vi "Read Target to Host FIFO.vi"(8 "error in (no error)":errorcluster) -> (0 "error out":errorcluster, 3 "Target to Host Data":u64[](array[numeric]))   [LabVIEW 2016]
uses:
  Host/Typedefs/IO Buffer Operation.ctl
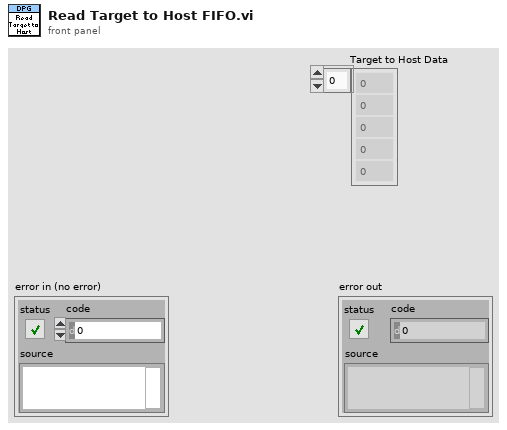
[diagram p1: front panel]
types:
  T1 = typedef "IO Buffer Operation.ctl" = enum16{"Initialize", "Write IO Data_Rd", "Read IO Data_Rd", "Write IO Data_Wr", "Read IO Data_Wr", "Write  IO Data_Dir", "Read  IO Data_Dir", "Write Host to Target FIFO", "Read Host to Target FIFO", "Write Target to Host FIFO", "Read Target to Host FIFO", "Write Monitor Enable?", "Read Monitor Enable?", "Close"}
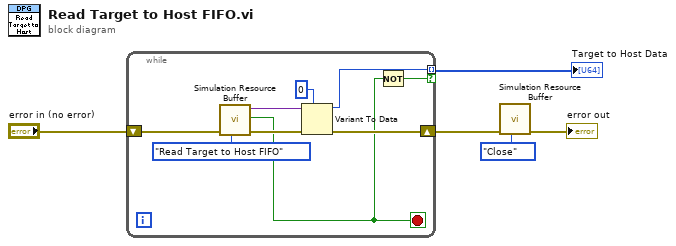
[diagram p0: block diagram]
diagram:
  n1 = while {
    tunnel: [w11] -> w5 mode=indexing if=w6
    shift-right: [w10] -> w4
    shift-left: "error in (no error)" -> [w9]
    stop <- w7 stop-if-true
    n2 = call "Simulation Resource Buffer.vi"("IO Buffer Operation"=IO_Buffer_Operation."Read Target to Host FIFO", "error in (no error)"=w9) -> ("error out"=w13:errorcluster, "Timed Out?"=w7:bool, "Data out"=w12:variant)  [unwired: 7 in]
    n3 = Variant To Data(error in=w13, type=u64 0 ("Target to Host Data"), Variant=w12) -> (data=w11:u64, error out=w10:errorcluster)
    n4 = Not(x=w7) -> (.not. x?=w6:bool)
  }
  "Target to Host Data" <- w5
  n5 = call "Simulation Resource Buffer.vi"("IO Buffer Operation"=IO_Buffer_Operation."Close", "error in (no error)"=w4) -> ("error out"=→"error out":errorcluster)  [unwired: 7 in, 2 out]
